vi "Write Database.vi"(8 "error in (no error)":errorcluster, 10 "Database.lvclass":refnum<class "Database.lvclass">, 11 "Form Configuration in":refnum<class "Form Model Configuration.lvclass">) -> (0 "error out":errorcluster, 3 "Form Configuration out":refnum<class "Form Model Configuration.lvclass">)   [LabVIEW 2020, in "Form Model Configuration.lvlib" / "Form Model Configuration.lvclass"]
uses:
  Form Model Configuration.lvclass
  source/Database/Database.lvclass
  Form Model Configuration.lvclass/Form Model Configuration.ctl
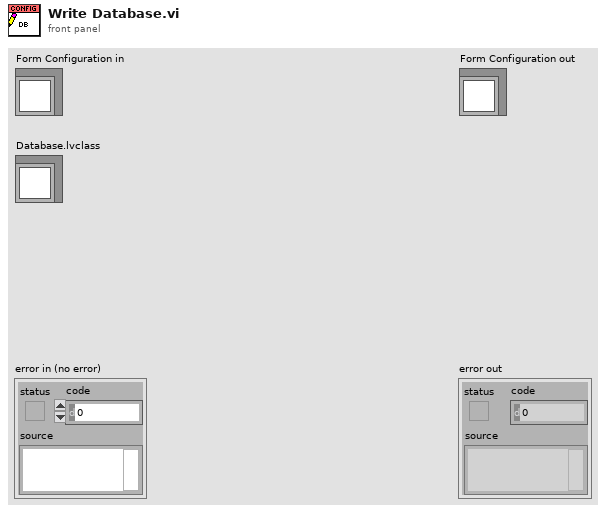
[diagram p1: front panel]
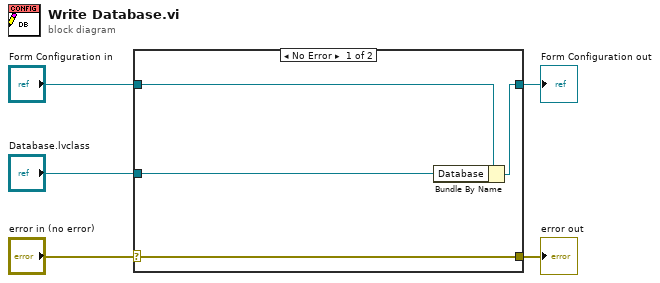
[diagram p0: block diagram]
diagram:
  n1 = case shown="No Error" "error in (no error)" {
    selector: "error in (no error)" -> [w9 w10]
    tunnel: [w9 w10] -> w4
    tunnel: [w7 w11] -> w2
    tunnel: "Form Configuration in" -> [w8 w11]
    tunnel: "Database.lvclass" -> [w6 _]
    frame No Error {
      n2 = Bundle By Name(cluster=w8, "Database"=w6) -> (w7:refnum<class "Form Model Configuration.lvclass">)
    }
    frame Error {
    }
  }
  "error out" <- w4
  "Form Configuration out" <- w2
